vi "Facade.vi"(0 "Data In":T4, 2 "Display State In":T2, 3 "Container State":T3) -> (6 "Data Out":T4, 7 "Display State Out":T2, 8 "Action":T1)   [LabVIEW 2015, in "KDemo.xctl"]
uses:
  KDemo.xctl
  Data.ctl
  KDemoBase Class/KDemoBase.lvclass
  <vilib>/_xctls/Container State.ctl
  State.ctl
  <vilib>/_xctls/Action.ctl
  KDemoBase Class/KDemoBase.lvclass/KDemoBase.ctl
  KDemoDerived Class/KDemoDerived.lvclass
  KDemoDerived Class/KDemoDerived.lvclass/KDemoDerived.ctl
  KDemoBase Class/Read Boolean.vi
  KDemoBase Class/Read Value.vi
  KDemoBase Class/Write Boolean.vi
  KDemoBase Class/Write Value.vi
  KDemoDerived Class/Write String.vi
  KDemoDerived Class/Read String.vi
  <vilib>/_xctls/XControlSupport.lvlib
  KObject Class/KObject.lvclass
panel:
  out "type-specific":bool
  in  "Type":u16(ring) items=["KDemoBase", "KDemoDerived"]
  in  "String":string
  in  "Value":dbl
  in  "Boolean":bool
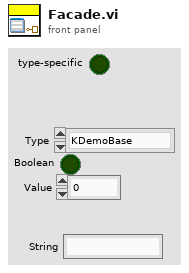
[diagram p1: front panel]
types:
  T1 = typedef "XControlSupport.lvlib/Action.ctl" = cluster{"Data Changed?":bool, "State Changed?":bool, "Action Name":string}
  T2 = typedef "KDemo.xctl/State.ctl" = cluster{"Numeric":dbl}
  T3 = typedef "XControlSupport.lvlib/Container State.ctl" = cluster{"Indicator?":bool, "Run Mode?":bool, " Refnum":refnum<vi>}
  T4 = typedef "KDemo.xctl/Data.ctl" = refnum<class "KDemoBase.lvclass">
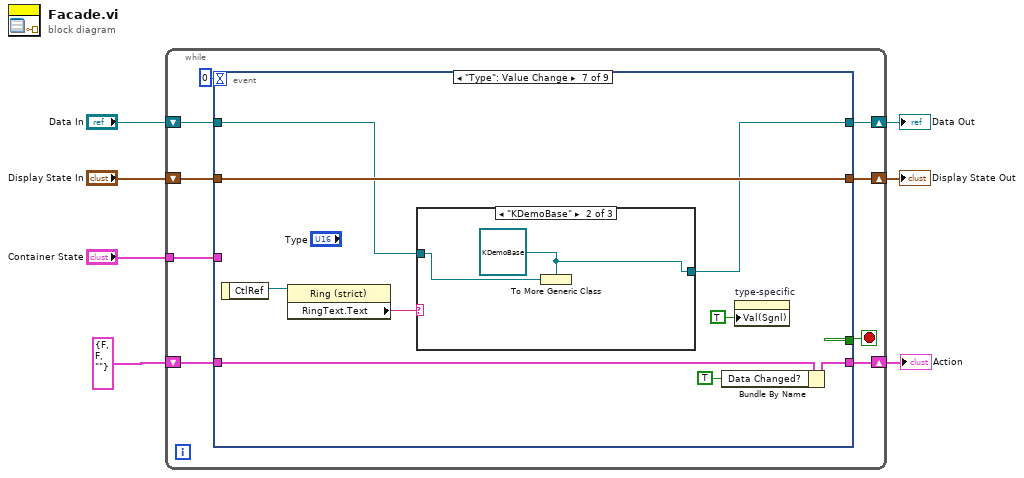
[diagram p0: block diagram]
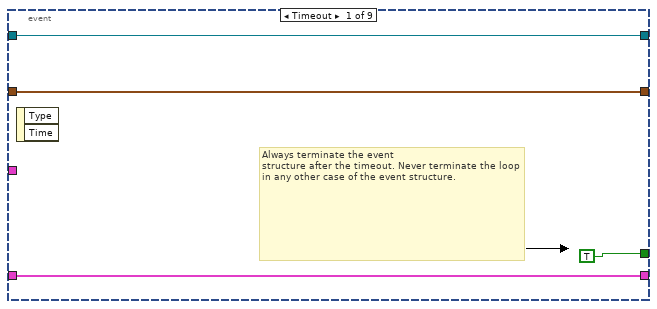
[diagram p2: hidden frame]
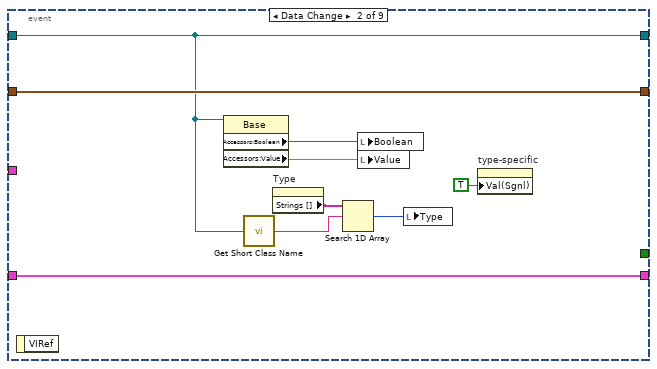
[diagram p3: hidden frame]
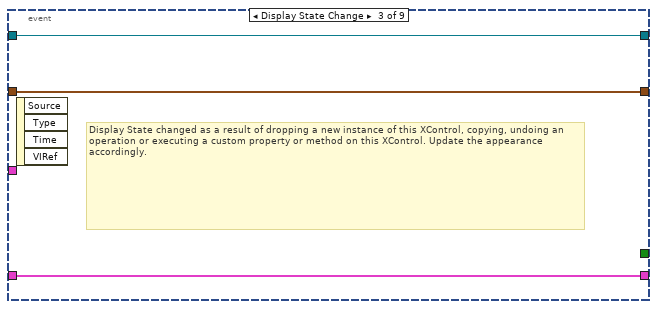
[diagram p4: hidden frame]
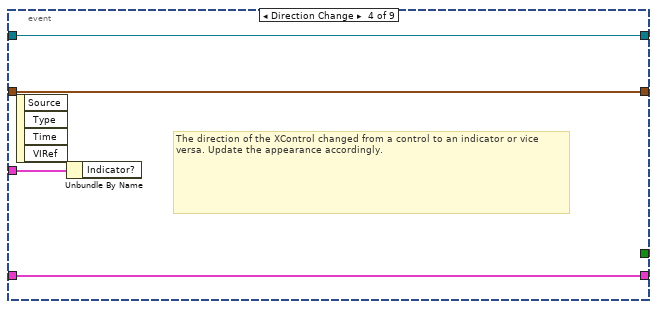
[diagram p5: hidden frame]
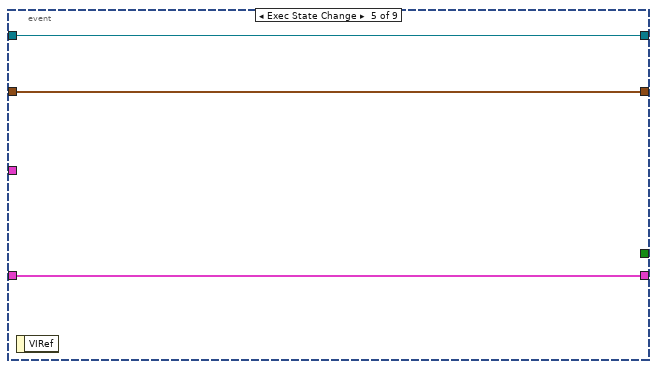
[diagram p6: hidden frame]
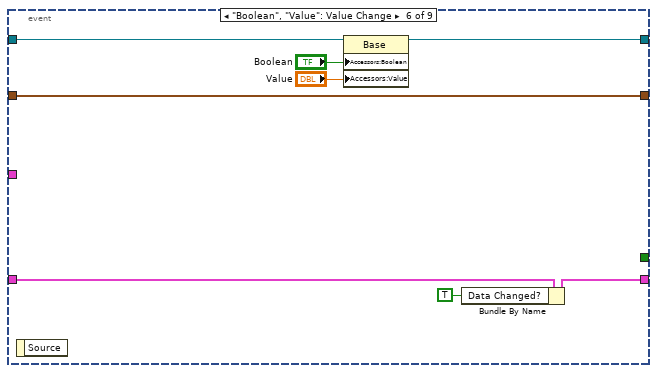
[diagram p7: hidden frame]
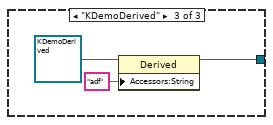
[diagram p9: hidden frame]
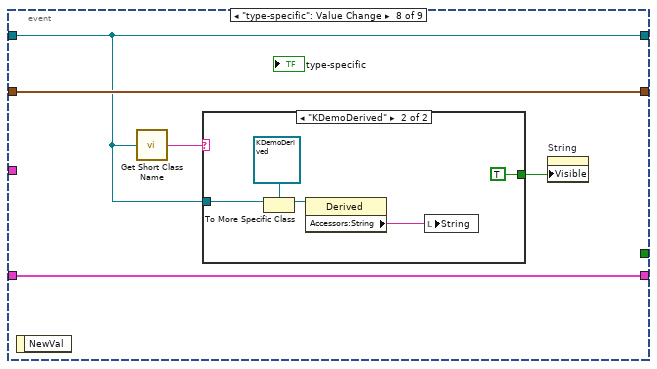
[diagram p10: hidden frame]
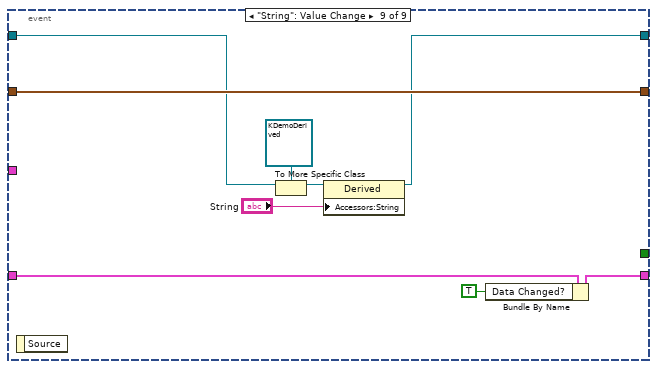
[diagram p12: hidden frame]
diagram:
  n1 = while {
    shift-right: [w15] -> w4
    shift-left: "Display State In" -> [w16]
    tunnel: "Container State" -> [w12]
    shift-right: [w10] -> w7
    shift-left: "Data In" -> [w11]
    shift-right: [w8] -> w2
    shift-left: T1 {"Data Changed?"=FALSE, "State Changed?"=FALSE, "Action Name"=""} ("Action") -> [w9]
    stop <- w14 stop-if-true
    n2 = event shown="[6] \"Type\": Value Change" {
      selector: _ -> [_ _ _ _ _ _ _ _ _]
      dyn-events: _ -> [_ _ _ _ _ _ _ _ _]
      timeout: 0 -> [_ _ _ _ _ _ _ _ _]
      tunnel: w16 -> [w18 w29 w32 w35 w39 w47 w56 w67 w81]
      tunnel: [w18 w29 w32 w35 w39 w47 w56 w67 w81] -> w15
      tunnel: [TRUE _ _ _ _ _ _ _ _] -> w14
      tunnel: w12 -> [_ _ _ w36 _ _ _ _ _]
      tunnel: w11 -> [w17 w24 w31 w34 w38 w46 w52 w64 w78]
      tunnel: [w17 w24 w31 w34 w38 w44 w51 w64 w75] -> w10
      tunnel: [w19 w28 w30 w33 w37 w41 w49 w66 w74] -> w8
      tunnel: w9 -> [w19 w28 w30 w33 w37 w45 w55 w66 w80]
      event Timeout {
        # "Always terminate the event\nstructure after the timeout. Never terminate the loop in any other case of the event structure."
        n3 = event-data() -> ()  [unwired: 1 in, 2 out]
      }
      event Data Change {
        n4 = event-data() -> ()  [unwired: 1 in, 1 out]
        n5 = property class="Base"(reference=w24) -> ("Accessors:Boolean"=w27:bool, "Accessors:Value"=w26:dbl)  [unwired: 1 in, 2 out]
        n6 = call "Get Short Class Name.vi"("KObject in"=w24) -> ("Class"=w23:string)  [unwired: 4 in]
        n7 = property on="Type" class="Ring (strict)"() -> ("Strings []"=w25:string[])  [unwired: 2 in, 2 out]
        n8 = Search 1D Array(1D array=w25, element=w23) -> (index of element=w22:i32)  [unwired: 1 in]
        n9 = local write "Boolean"(w27) -> ()
        n10 = local write "Value"(w26) -> ()
        n11 = local write "Type"(w22) -> ()
        n12 = property on="type-specific" class="Bool (strict)"("Val(Sgnl)"=TRUE ("Value (Signaling)")) -> ()  [unwired: 2 in, 2 out]
      }
      event Display State Change {
        # "Display State changed as a result of dropping a new instance of this XControl, copying, undoing an operation or executing a custom property or method on this XControl. Update the appearance accordingly."
        n13 = event-data() -> ()  [unwired: 1 in, 4 out]
      }
      event Direction Change {
        # "The direction of the XControl changed from a control to an indicator or vice versa. Update the appearance accordingly."
        n14 = event-data() -> ()  [unwired: 1 in, 4 out]
        n15 = Unbundle By Name(w36) -> ()  [unwired: 1 out]
      }
      event Exec State Change {
        n16 = event-data() -> ()  [unwired: 1 in, 1 out]
      }
      event "Boolean", "Value": Value Change {
        n17 = event-data() -> ()  [unwired: 1 in, 1 out]
        n18 = property class="Base"(reference=w46, "Accessors:Boolean"="Boolean", "Accessors:Value"="Value") -> (reference out=w44:T4)  [unwired: 1 in, 1 out]
        n19 = Bundle By Name(cluster=w45, "Data Changed?"=TRUE) -> (w41:T1)
      }
      event "Type": Value Change {
        n20 = event-data() -> ("CtlRef"=w54:refnum<vi>)  [unwired: 1 in]
        n21 = property class="Ring (strict)"(reference=w54) -> ("RingText.Text"=w53:string)  [unwired: 1 in, 2 out]
        n22 = case shown="\"KDemoBase\"" w53 {
          tunnel: w52 -> [w57 w59 _]
          tunnel: [w57 w58 w60] -> w51
          frame "False", Default {
          }
          frame "KDemoBase" {
            w58 = T4 refnum ("Data In")
            n23 = To More Generic Class(target class=w58, reference=w59) -> ()  [unwired: 1 out]
          }
          frame "KDemoDerived" {
            n24 = property class="Derived"(reference=refnum<class "KDemoDerived.lvclass"> refnum ("Gen2"), "Accessors:String"="adf" ("String")) -> (reference out=w60:refnum<class "KDemoDerived.lvclass">)  [unwired: 1 in, 1 out]
          }
        }
        n25 = Bundle By Name(cluster=w55, "Data Changed?"=TRUE) -> (w49:T1)
        n26 = property on="type-specific" class="Bool (strict)"("Val(Sgnl)"=TRUE ("Value (Signaling)")) -> ()  [unwired: 2 in, 2 out]
      }
      event "type-specific": Value Change {
        n27 = event-data() -> ()  [unwired: 1 in, 1 out]
        n28 = call "Get Short Class Name.vi"("KObject in"=w64) -> ("Class"=w65:string)  [unwired: 4 in]
        n29 = case shown="\"KDemoDerived\"" w65 {
          tunnel: w64 -> [_ w71]
          tunnel: [_ TRUE] -> w63
          frame "False", Default {
          }
          frame "KDemoDerived" {
            n30 = To More Specific Class(target class=refnum<class "KDemoDerived.lvclass"> refnum ("Gen2"), reference=w71) -> (specific class reference=w70:refnum<class "KDemoDerived.lvclass">)  [unwired: 1 in, 1 out]
            n31 = property class="Derived"(reference=w70) -> ("Accessors:String"=w69:string)  [unwired: 1 in, 2 out]
            n32 = local write "String"(w69) -> ()
          }
        }
        n33 = property on="String" class="Str"("Visible"=w63) -> ()  [unwired: 2 in, 2 out]
      }
      event "String": Value Change {
        n34 = event-data() -> ()  [unwired: 1 in, 1 out]
        n35 = To More Specific Class(target class=refnum<class "KDemoDerived.lvclass"> refnum ("Gen2"), reference=w78) -> (specific class reference=w77:refnum<class "KDemoDerived.lvclass">)  [unwired: 1 in, 1 out]
        n36 = property class="Derived"(reference=w77, "Accessors:String"="String") -> (reference out=w75:refnum<class "KDemoDerived.lvclass">)  [unwired: 1 in, 1 out]
        n37 = Bundle By Name(cluster=w80, "Data Changed?"=TRUE) -> (w74:T1)
      }
    }
  }
  "Display State Out" <- w4
  "Data Out" <- w7
  "Action" <- w2
